vi "PID Gyro.vi"(6 "K_i":sgl=0.0014, 7 "K_p":sgl=0.6, 9 "Previous integral":sgl, 10 "Target angle":sgl, 11 "EV3 in":T1) -> (1 "New integral":sgl, 2 "Total error":sgl, 3 "EV3 out":T1)   [LabVIEW 2016]
uses:
  <vilib>/NXT/Subs/LVHSConnector.ctl
  <vilib>/NXT/LegoClasses/BrickReference/BrickReference.lvclass
  <vilib>/NXT/Block Support/NXT_InputPort.ctl
  <vilib>/NXT/Dual Mode Library/Sensors/EV3_Gyro_Angle.vi
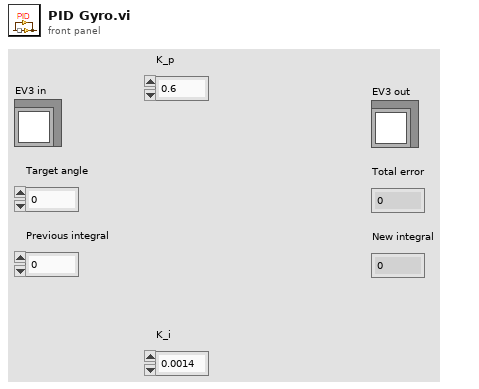
[diagram p1: front panel]
types:
  T1 = typedef "LVHSConnector.ctl" = refnum<class "BrickReference.lvclass">
  T2 = typedef "NXT_InputPort.ctl" = u32
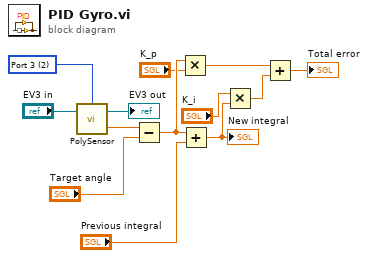
[diagram p0: block diagram]
diagram:
  w13 = T2 2 items=["Port 1", "Port 2", "Port 3", "Port 4"] ("Port (Gyro)")
  n1 = call-poly <vilib>:"PolySensor.vi"("NXT/EV3"="EV3 in", "Port (Port 1)"=w13) -> ("Degrees"=w1:sgl, "NXT/EV3"=→"EV3 out":T1)  [unwired: 1 in]
  n2 = Subtract(x=w1, y="Target angle") -> (x-y=w9:sgl)
  n3 = Multiply(x=w9, y="K_p") -> (x*y=w6:sgl)
  n4 = Add(x=w9, y="Previous integral") -> (x+y=w4:sgl)
  "New integral" <- w4
  n5 = Multiply(x="K_i", y=w4) -> (x*y=w7:sgl)
  n6 = Add(x=w6, y=w7) -> (x+y=→"Total error":sgl)
